vi "svl_Check Exp Mode and Time Constant.vi"(4 "time constant [ms]":dbl format="%.2f", 6 "exponential mode":enum16{"Slow", "Fast", "Impulse", "Custom"}(ring), 8 "error in (no error)":errorcluster) -> (0 "error out":errorcluster, 1 "parameter has changed":bool)   [LabVIEW 2017]
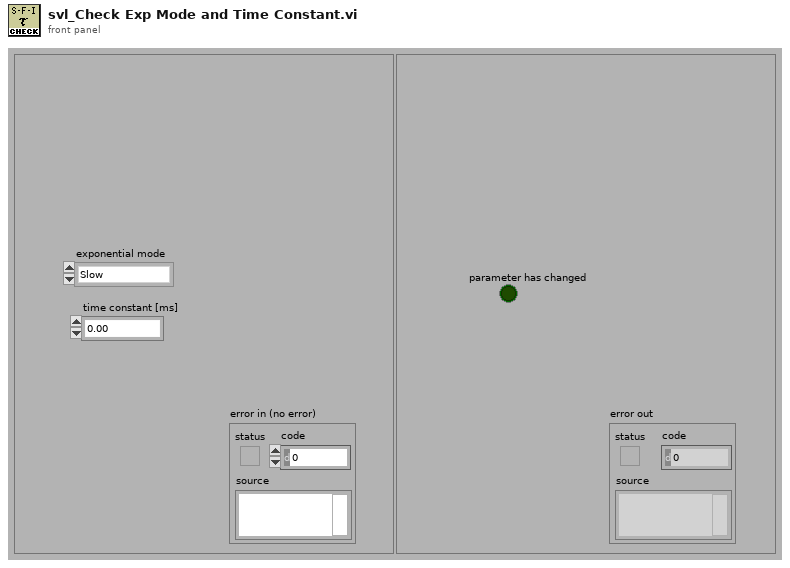
[diagram p1: front panel]
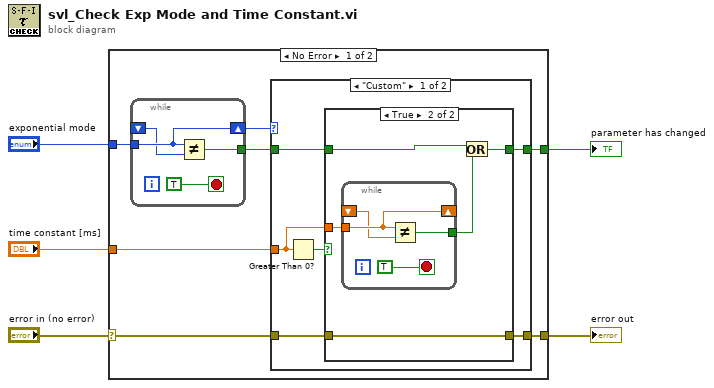
[diagram p0: block diagram]
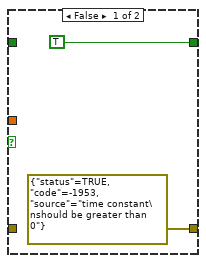
[diagram p2: hidden frame]
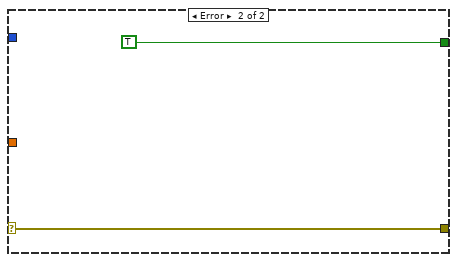
[diagram p4: hidden frame]
diagram:
  n1 = case shown="No Error" "error in (no error)" {
    selector: "error in (no error)" -> [w10 w37]
    tunnel: [w7 TRUE] -> w5
    tunnel: "exponential mode" -> [w12 _]
    tunnel: [w9 w37] -> w2
    tunnel: "time constant [ms]" -> [w6 _]
    frame No Error {
      n2 = while {
        tunnel: [w13] -> w8
        tunnel: w12 -> [w15]
        shift-left: _ -> [w14]
        shift-right: [w15] -> w11
        stop <- TRUE stop-if-true
        n3 = Not Equal?(x=w15, y=w14) -> (x != y?=w13:bool)
      }
      n4 = case shown="\"Custom\"" w11 {
        tunnel: w10 -> [w20 w35]
        tunnel: [w17 w35] -> w9
        tunnel: [w22 w34] -> w7
        tunnel: w8 -> [w18 w34]
        tunnel: w6 -> [w19 _]
        frame "Custom" {
          n5 = Greater Than 0?(x=w19) -> (x > 0?=w21:bool)
          n6 = case shown="True" w21 {
            tunnel: [TRUE w26] -> w22
            tunnel: [errorcluster {"status"=TRUE, "code"=-1953, "source"="time constant\nshould be greater than 0"} ("error IO") w25] -> w17
            tunnel: w20 -> [_ w25]
            tunnel: w19 -> [_ w29]
            tunnel: w18 -> [_ w28]
            frame False {
            }
            frame True {
              n7 = while {
                tunnel: w29 -> [w31]
                tunnel: [w32] -> w27
                shift-left: _ -> [w30]
                shift-right: [w31] -> _
                stop <- TRUE stop-if-true
                n8 = Not Equal?(x=w31, y=w30) -> (x != y?=w32:bool)
              }
              n9 = Or(x=w28, y=w27) -> (x .or. y?=w26:bool)
            }
          }
        }
        frame "Slow".."Impulse", Default {
        }
      }
    }
    frame Error {
    }
  }
  "parameter has changed" <- w5
  "error out" <- w2
